vi "cDAQ to PC fglbl.vi"(5 "message":T4, 7 "PC HMI Thread":T5, 8 "error in (no error)":errorcluster, 10 "tcp connection info":T1, 11 "action":T3) -> (0 "error out":errorcluster)   [LabVIEW 2012]
uses:
  interthread comms/typedefs/station cDAQ thread IDs.ctl
  interthread comms/typedefs/state queue fglbl actions.ctl
  interthread comms/typedefs/interthread message.ctl
  typedefs/connection type.ctl
  typedefs/tcp connection info.ctl
  interthread comms/typedefs/app type.ctl
  typedefs/interapp tx message request.ctl
  interthread comms/typedefs/HMI PC thread IDs.ctl
  typedefs/interapp message actions.ctl
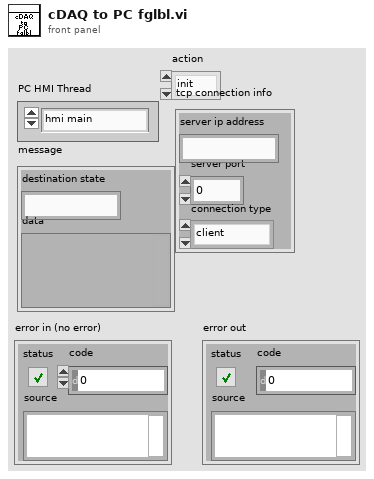
[diagram p1: front panel]
types:
  T1 = typedef "tcp connection info.ctl" = cluster{"server ip address":string, "server port":i32, "connection type":T2}
  T2 = typedef "connection type.ctl" = enum16{"client", "server"}
  T3 = typedef "interapp message actions.ctl" = enum16{"init", "request message tx"}
  T4 = typedef "interthread message.ctl" = cluster{"destination state":string, "data":variant}
  T5 = typedef "HMI PC thread IDs.ctl" = enum16{"hmi main", "file output", "tcp comms", "NVH process"}
  T6 = typedef "app type.ctl" = enum16{"PC", "cDAQ", "AuditHMI"}
  T7 = typedef "interapp tx message request.ctl" = cluster{"destination app":T6, "destination thread":string, "tcp connection info":T1, "message":T4}
  T8 = typedef "state queue fglbl actions.ctl" = enum16{"init queues", "get queue ref", "destroy queues"}
  T9 = typedef "station cDAQ thread IDs.ctl" = enum16{"cDAQ main", "analog input", "eol test exe", "nvh test exe", "tcp comms"}
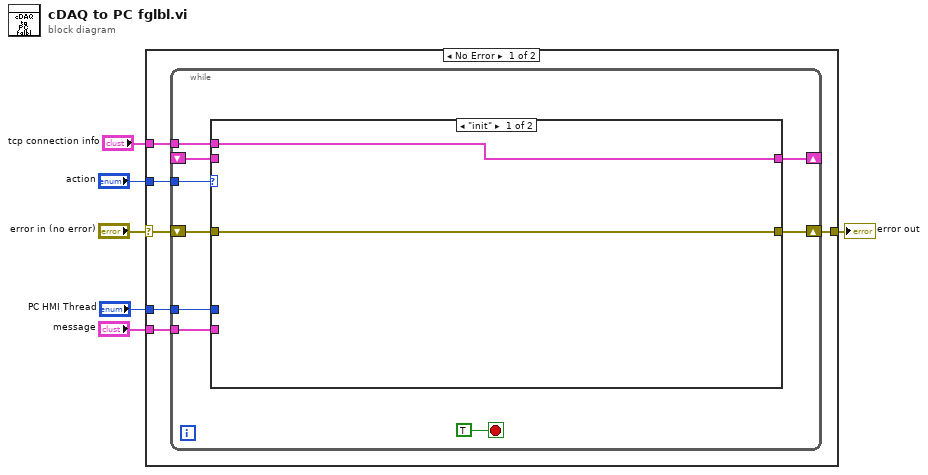
[diagram p0: block diagram]
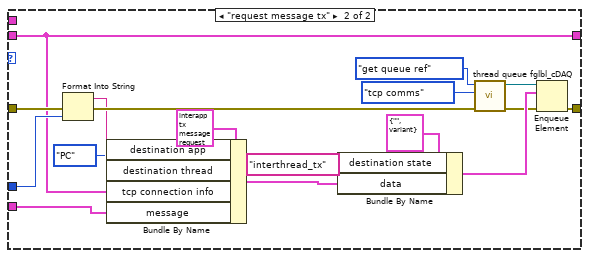
[diagram p2: hidden frame]
diagram:
  n1 = case shown="No Error" "error in (no error)" {
    selector: "error in (no error)" -> [w9 w41]
    tunnel: [w12 w41] -> w6
    tunnel: "PC HMI Thread" -> [w11 _]
    tunnel: "message" -> [w10 _]
    tunnel: "action" -> [w8 _]
    tunnel: "tcp connection info" -> [w7 _]
    frame No Error {
      n2 = while {
        tunnel: w11 -> [w20]
        tunnel: w10 -> [w19]
        shift-right: [w21] -> w12
        shift-left: w9 -> [w18]
        tunnel: w8 -> [w16]
        shift-right: [w14] -> _
        shift-left: _ -> [w13]
        tunnel: w7 -> [w15]
        stop <- TRUE stop-if-true
        n3 = case shown="\"init\"" w16 {
          tunnel: [w22 w40] -> w21
          tunnel: w20 -> [_ w37]
          tunnel: w19 -> [_ w35]
          tunnel: w18 -> [w22 w25]
          tunnel: w15 -> [w23 _]
          tunnel: [w23 w24] -> w14
          tunnel: w13 -> [_ w24]
          frame "init" {
          }
          frame "request message tx" {
            n4 = Format Into String(error in=w25, w37) -> (resulting string=w38:string, error out=w39:errorcluster)  [unwired: 2 in]
            n5 = Bundle By Name(cluster=T7 {"destination app"=enum."PC", "destination thread"="", "tcp connection info"={"server ip address"="", "server port"=0, "connection type"=enum."client"}, "message"={"destination state"="", "data"=variant}}, "destination app"=app_type."PC", "destination thread"=w38, "tcp connection info"=w24, "message"=w35) -> (w34:T7)
            n6 = Bundle By Name(cluster=T4 {"destination state"="", "data"=variant} ("message"), "destination state"="interthread_tx", "data"=w34) -> (w32:T4)
            n7 = call "thread queue fglbl_cDAQ.vi"("error in (no error)"=w39, "Station cDAQ Thread Queue"=station_cDAQ_thread_IDs."tcp comms", "action"=state_queue_fglbl_actions."get queue ref") -> ("error out"=w28:errorcluster, "queue out"=w29:refnum<queue>)  [unwired: 6 in, 1 out]
            n8 = Enqueue Element(queue=w29, element=w32, error in (no error)=w28) -> (error out=w40:errorcluster)  [unwired: 1 in, 2 out]
          }
        }
      }
    }
    frame Error {
    }
  }
  "error out" <- w6
